vi "Prepend Changed Item Names.vi"(11 "VI Data in":T1[](array[typedef])) -> (3 "Array":string[](array[string]))   [LabVIEW 2023, in "VI Properties Editor.lvlib"]
uses:
  VI Properties Editor.lvlib
  CTLs/VI Data.ctl
  <vilib>/picture/picture.llb/imagedata.ctl
  CTLs/VI Properties.ctl
  CTLs/Control Properties.ctl
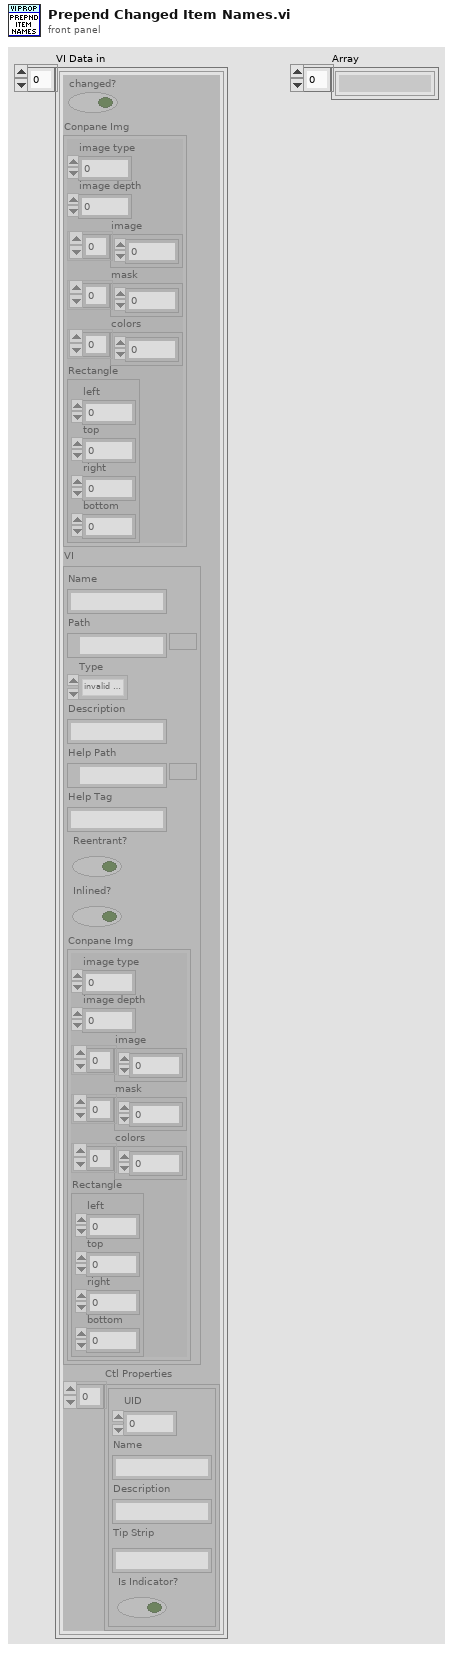
[diagram p1: front panel]
types:
  T1 = typedef "VI Properties Editor.lvlib/VI Data.ctl" = cluster{"changed?":bool, "Conpane Img":T2, "VI":T3, "Ctl Properties":T4[]}
  T2 = typedef "imagedata.ctl" = cluster{"image type":i32, "image depth":i32, "image":u8[], "mask":u8[], "colors":u32[], "Rectangle":cluster{"left":i16, "top":i16, "right":i16, "bottom":i16}}
  T3 = typedef "VI Properties Editor.lvlib/VI Properties.ctl" = cluster{"Name":string, "Path":path, "Type":enum32{"invalid VI type", "Standard VI", "Control VI", "Global VI", "Polymorphic VI", "Configuration VI", "SubSystem", "Facade VI", "Method VI", "Statechart Diagram VI"}, "Description":string, "Help Path":path, "Help Tag":string, "Reentrant?":bool, "Inlined?":bool, "Conpane Img":T2}
  T4 = typedef "VI Properties Editor.lvlib/Control Properties.ctl" = cluster{"UID":i32, "Name":string, "Description":string, "Tip Strip":string, "Is Indicator?":bool}
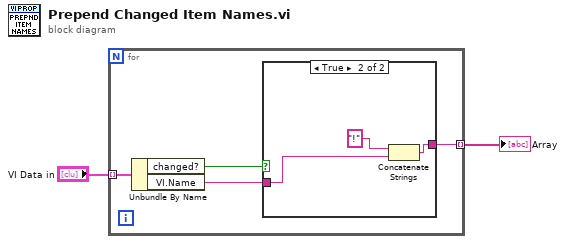
[diagram p0: block diagram]
diagram:
  n1 = for {
    tunnel: "VI Data in" -> [w6] mode=indexing
    tunnel: [w5] -> w2 mode=indexing
    n2 = Unbundle By Name(w6) -> ("changed?"=w4:bool, "VI.Name"=w3:string)
    n3 = case shown="True" w4 {
      tunnel: [w7 w10] -> w5
      tunnel: w3 -> [w7 w9]
      frame False {
      }
      frame True {
        n4 = Concatenate Strings("!" ("format string"), w9) -> (w10:string)
      }
    }
  }
  "Array" <- w2
